vi "Get Number of Elements.vi"(8 "error in (no error)":errorcluster, 10 "Size Info":T1, 11 "CIPC Reference":u64) -> (0 "error out":errorcluster, 2 "elements_lost":u32, 3 "elements_available":u32)   [LabVIEW 2021, in "CIF_NI_CIPC.lvlib"]
doc: "Check the number of elements available in the buffer.\n\nOutputs:\n- elements_available: number of elements which can still be read from the buffer\n- elements_missed: number of elements which were missed and cannot be read anymore (since the memory was overwritten)"
uses:
  CIF_NI_CIPC.lvlib
  TypeDefs/Info Size.ctl
  SubVIs/Check Error.vi
  <vilib>/Utility/error.llb/Trim Whitespace.vi
  <vilib>/Utility/error.llb/Error Cluster From Error Code.vi
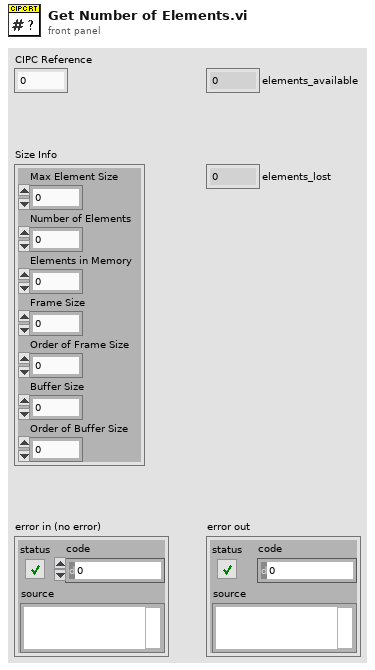
[diagram p1: front panel]
types:
  T1 = typedef "CIF_NI_CIPC.lvlib/Info Size.ctl" = cluster{"Max Element Size":u32, "Number of Elements":u32, "Elements in Memory":u32, "Frame Size":u32, "Order of Frame Size":u32, "Buffer Size":u32, "Order of Buffer Size":u32}
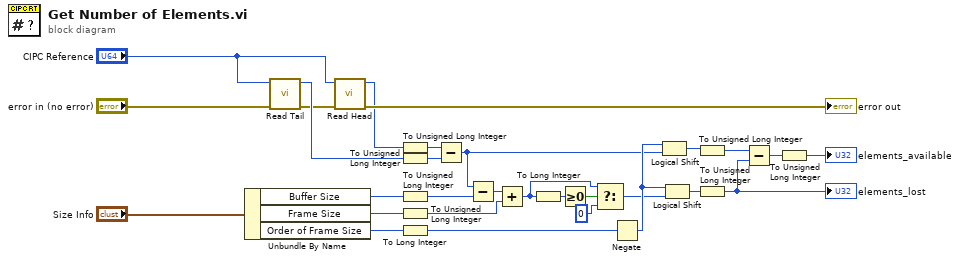
[diagram p0: block diagram]
diagram:
  n1 = Unbundle By Name("Size Info") -> ("Buffer Size"=w14:u32, "Frame Size"=w11:u32, "Order of Frame Size"=w1:u32)
  n2 = call "Read Tail.vi"("error in (no error)"="error in (no error)", "CIPC Reference"="CIPC Reference") -> ("error out"=w7:errorcluster, "Tail"=w8:u32)  [unwired: 8 in]
  n3 = call "Read Head.vi"("error in (no error)"=w7, "CIPC Reference"="CIPC Reference") -> ("error out"=→"error out":errorcluster, "Head"=w22:u32)  [unwired: 8 in]
  n4 = To Unsigned Long Integer(number=w22) -> (unsigned 32bit integer=w23:u32)
  n5 = To Unsigned Long Integer(number=w8) -> (unsigned 32bit integer=w24:u32)
  n6 = To Unsigned Long Integer(number=w14) -> (unsigned 32bit integer=w18:u32)
  n7 = To Unsigned Long Integer(number=w11) -> (unsigned 32bit integer=w10:u32)
  n8 = To Long Integer(number=w1) -> (32bit integer=w29:i32)
  n9 = Subtract(x=w23, y=w24) -> (x-y=w19:u32)
  n10 = Subtract(x=w19, y=w18) -> (x-y=w12:u32)
  n11 = Add(x=w12, y=w10) -> (x+y=w9:u32)
  n12 = To Long Integer(number=w9) -> (32bit integer=w17:i32)
  n13 = Greater Or Equal To 0?(x=w17) -> (x >= 0?=w16:bool)
  n14 = Select(t=w9, s=w16, f=u32 0) -> (s? t:f=w13:u32)
  n15 = Negate(x=w29) -> (-x=w20:i32)
  n16 = Logical Shift(y=w20, x=w19) -> (x << y=w21:u32)
  n17 = Logical Shift(y=w20, x=w13) -> (x << y=w27:u32)
  n18 = To Unsigned Long Integer(number=w21) -> (unsigned 32bit integer=w26:u32)
  n19 = To Unsigned Long Integer(number=w27) -> (unsigned 32bit integer=w25:u32)
  "elements_lost" <- w25
  n20 = Subtract(x=w26, y=w25) -> (x-y=w3:u32)
  n21 = To Unsigned Long Integer(number=w3) -> (unsigned 32bit integer=→"elements_available":u32)
